vi "Del Data OD reference.vi"(8 "error in (no error)":errorcluster, 11 "Experiment in":refnum<class "Experiment.lvclass">) -> (0 "error out":errorcluster, 3 "Experiment out":refnum<class "Experiment.lvclass">)   [LabVIEW 2015, in "Experiment.lvclass"]
uses:
  Experiment.lvclass
  Experiment.lvclass/Experiment.ctl
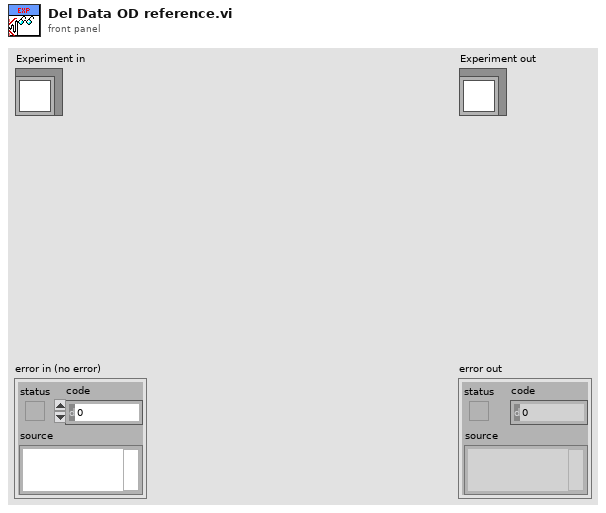
[diagram p1: front panel]
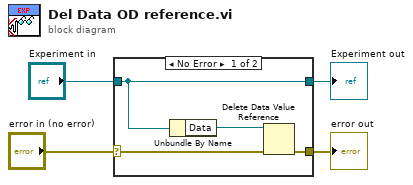
[diagram p0: block diagram]
diagram:
  n1 = case shown="No Error" "error in (no error)" {
    selector: "error in (no error)" -> [w5 w9]
    tunnel: [w6 w9] -> w3
    tunnel: [w8 w10] -> w1
    tunnel: "Experiment in" -> [w8 w10]
    frame No Error {
      n2 = Unbundle By Name(w8) -> ("Data"=w7:refnum<data-value>)
      n3 = Delete Data Value Reference(data value reference=w7, error in=w5) -> (error out=w6:errorcluster)  [unwired: 1 out]
    }
    frame Error {
    }
  }
  "error out" <- w3
  "Experiment out" <- w1
